vi "SpinCounter.vi"(11 "WheelSpins":dbl) -> ()   [LabVIEW 2019]
panel:
  out "EighthCycles":dbl
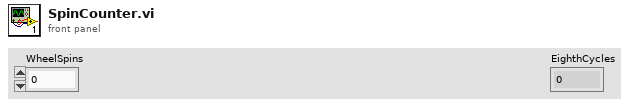
[diagram p1: front panel]
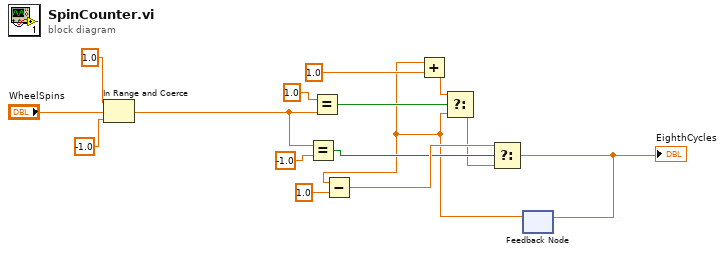
[diagram p0: block diagram]
diagram:
  n1 = In Range and Coerce(upper limit=1.0, x="WheelSpins", lower limit=-1.0) -> (coerced(x)=w3:dbl)  [unwired: 1 out]
  n2 = Equal?(x=w3, y=-1.0) -> (x = y?=w7:bool)
  n3 = Equal?(x=1.0, y=w3) -> (x = y?=w12:bool)
  n4 = feedback #1() -> (w4:dbl)  [unwired: 1 in]
  n5 = Subtract(x=w4, y=1.0) -> (x-y=w8:dbl)
  n6 = Add(x=w4, y=1.0) -> (x+y=w11:dbl)
  n7 = Select(t=w11, s=w12, f=w4) -> (s? t:f=w6:dbl)
  n8 = Select(t=w8, s=w7, f=w6) -> (s? t:f=w5:dbl)
  "EighthCycles" <- w5
  n9 = feedback-in #1(w5) -> ()
